vi "connect in_FPGA.vi"(6 "error in (no error)":errorcluster) -> (0 "error out":errorcluster, 3 "Database Connection":T1, 9 "Test Server":bool)   [LabVIEW 2012]
uses:
  <vilib>/addons/database/Connection.llb/Conn ObjectReference.ctl
  <vilib>/addons/database/Connection.llb/DB Tools Open Connec (String).vi
  <vilib>/addons/database/NI_Database_API.lvlib
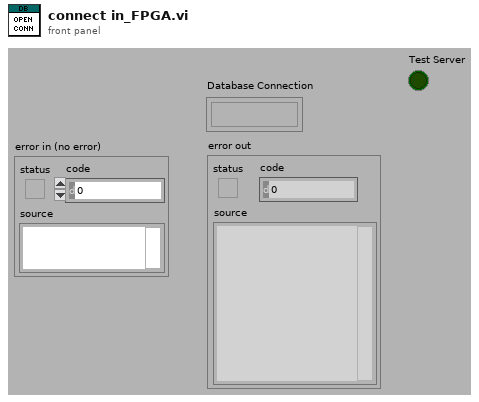
[diagram p1: front panel]
types:
  T1 = typedef "NI_Database_API.lvlib/Conn ObjectReference.ctl" = refnum<k1>
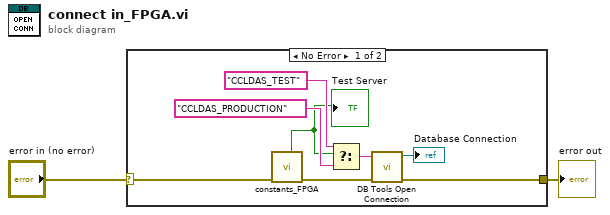
[diagram p0: block diagram]
diagram:
  n1 = case shown="No Error" "error in (no error)" {
    selector: "error in (no error)" -> [w4 w11]
    tunnel: [w9 w11] -> w1
    frame No Error {
      n2 = call "constants_FPGA.vi"("error in (no error)"=w4) -> ("error out"=w3:errorcluster, "Testing"=w5:bool)  [unwired: 4 in, 5 out]
      "Test Server" <- w5
      n3 = Select(t="CCLDAS_TEST", s=w5, f="CCLDAS_PRODUCTION") -> (s? t:f=w6:string)
      n4 = call-poly <vilib>:"DB Tools Open Connection.vi"("error in (no error)"=w3, "connection information"=w6) -> ("error out"=w9:errorcluster, "connection reference"=→"Database Connection":T1)  [unwired: 6 in]
    }
    frame Error {
    }
  }
  "error out" <- w1
